vi "read parameters in a cluster from last configuration file.vi"(8 "error in (no error)":errorcluster, 9 "Control in":refnum<vi>, 10 "section":string, 11 "refnum in":T1) -> (0 "error out":errorcluster, 3 "Refnum out":T1)   [LabVIEW 2015]
uses:
  <vilib>/Utility/config.llb/Config Data RefNum.ctl
  <vilib>/Utility/config.llb/Read Key (String).vi
  <vilib>/Utility/config.llb/Read Key (Double).vi
  <vilib>/Utility/config.llb/Read Key (Boolean).vi
  <vilib>/Utility/config.llb/NI_LVConfig.lvlib
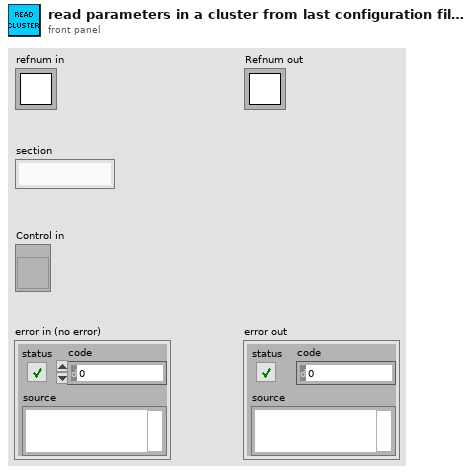
[diagram p1: front panel]
types:
  T1 = typedef "NI_LVConfig.lvlib/Config Data RefNum.ctl" = refnum<k1>
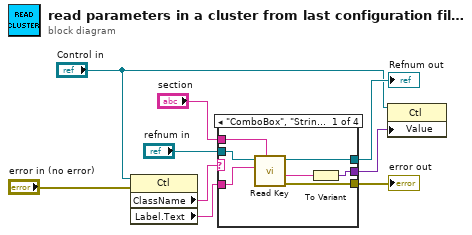
[diagram p0: block diagram]
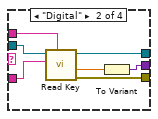
[diagram p2: hidden frame]
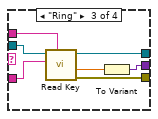
[diagram p3: hidden frame]
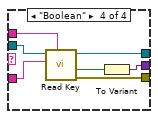
[diagram p4: hidden frame]
diagram:
  n1 = property class="Ctl"(reference="Control in", error in="error in (no error)") -> ("ClassName"=w3:string, "Label.Text"=w5:string)  [unwired: 2 out]
  n2 = case shown="\"ComboBox\", \"String\", Default" w3 {
    tunnel: "refnum in" -> [w16 w23 w30 w37]
    tunnel: w5 -> [w15 w22 w29 w36]
    tunnel: "section" -> [w14 w21 w28 w35]
    tunnel: [w12 w19 w26 w33] -> w7
    tunnel: [w11 w18 w25 w32] -> w9
    tunnel: [w10 w17 w24 w31] -> w1
    frame "ComboBox", "String", Default {
      n3 = call-poly <vilib>:"Read Key.vi"("section"=w14, "key"=w15, "refnum"=w16) -> ("error out"=w10:errorcluster, "value"=w13:string, "refnum out"=w11:T1)  [unwired: 5 in, 1 out]
      n4 = To Variant(anything=w13) -> (Variant=w12:variant)
    }
    frame "Digital" {
      n5 = call-poly <vilib>:"Read Key.vi"("section"=w21, "key"=w22, "refnum"=w23) -> ("error out"=w17:errorcluster, "value"=w20:dbl, "refnum out"=w18:T1)  [unwired: 5 in, 1 out]
      n6 = To Variant(anything=w20) -> (Variant=w19:variant)
    }
    frame "Ring" {
      n7 = call-poly <vilib>:"Read Key.vi"("section"=w28, "key"=w29, "refnum"=w30) -> ("error out"=w24:errorcluster, "value"=w27:dbl, "refnum out"=w25:T1)  [unwired: 5 in, 1 out]
      n8 = To Variant(anything=w27) -> (Variant=w26:variant)
    }
    frame "Boolean" {
      n9 = call-poly <vilib>:"Read Key.vi"("section"=w35, "key"=w36, "refnum"=w37) -> ("error out"=w31:errorcluster, "value"=w34:bool, "refnum out"=w32:T1)  [unwired: 5 in, 1 out]
      n10 = To Variant(anything=w34) -> (Variant=w33:variant)
    }
  }
  "Refnum out" <- w9
  "error out" <- w1
  n11 = property class="Ctl"(reference="Control in", "Value"=w7) -> ()  [unwired: 1 in, 2 out]
